vi "CPLX_SGL.vi"(4 "Value":csg) -> (1 "Constant":refnum<class "Abs_Complex Single Float.lvclass">)   [LabVIEW 2021, in "Const_CPLX_SGL.lvclass"]
uses:
  Const_CPLX_SGL.lvclass
  Abs_Types/Complex Single Float/Abs_Complex Single Float.lvclass
  C:/Program Files (x86)/National Instruments/LabVIEW 2021/vi.lib/TSA/Abstract Data Classes/Abs_Types/Complex Single Float/Abs_Complex Single Float.lvclass
  Const_CPLX_SGL.lvclass/Const_CPLX_SGL.ctl
  Properties/Write Value.vi
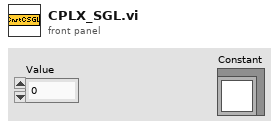
[diagram p1: front panel]
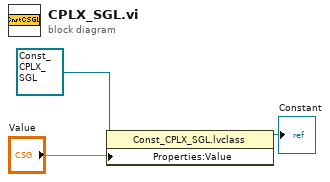
[diagram p0: block diagram]
diagram:
  n1 = property class="Const_CPLX_SGL.lvclass"(reference=refnum<class "Const_CPLX_SGL.lvclass"> refnum ("Constants.lvlib:Numeric.lvclass"), "Properties:Value"="Value") -> (reference out=→"Constant":refnum<class "Const_CPLX_SGL.lvclass">)  [unwired: 1 in, 1 out]
